vi "get all FPGA CD resources.vi"(7 "Show":T1, 8 "error in (no error)":errorcluster, 11 "Item Ref in":T3 format="%.0x") -> (0 "error out":errorcluster, 2 "resource entries":T2[](array[typedef]) {"FPGA CD Ref" format="%.0x"; "reserver" format="%.0x"}, 3 "Item Ref out":T3 format="%.0x")   [LabVIEW 2016, in "FPGA Resource Manager.lvlib"]
uses:
  FPGA Resource Manager.lvlib
  <vilib>/NI Veristand/Custom Device API/Custom Device Item Ref.ctl
  resource info.ctl
  viz_show.ctl
  <vilib>/NI VeriStand/Custom Device API/Custom Device API.lvlib
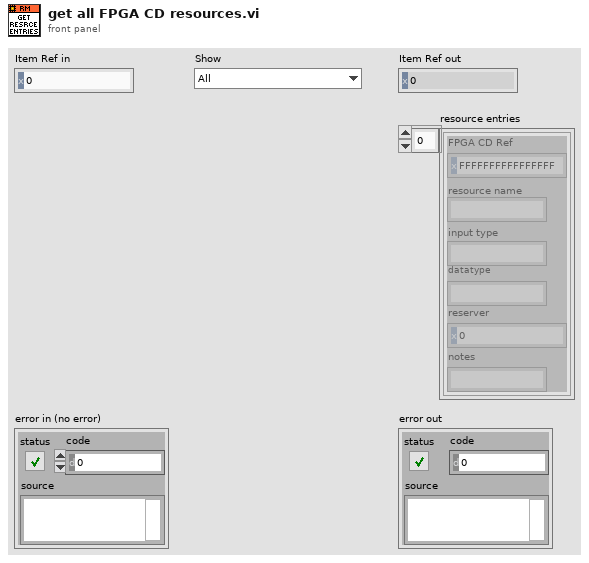
[diagram p1: front panel]
types:
  T1 = typedef "FPGA Resource Manager.lvlib/viz_show.ctl" = enum16{"All", "Mapped", "Unmapped"}
  T2 = typedef "FPGA Resource Manager.lvlib/resource info.ctl" = cluster{"FPGA CD Ref":T3, "resource name":string, "input type":string, "datatype":string, "reserver":T3, "notes":string}
  T3 = typedef "Custom Device API.lvlib/Custom Device Item Ref.ctl" = u64
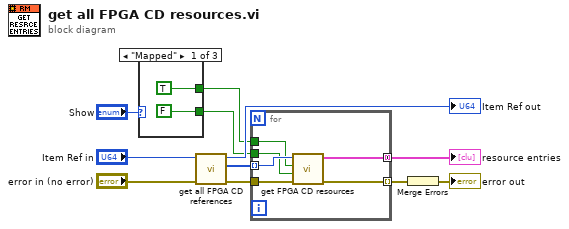
[diagram p0: block diagram]
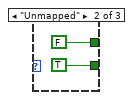
[diagram p2: hidden frame]
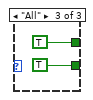
[diagram p3: hidden frame]
diagram:
  n1 = case shown="\"Mapped\"" "Show" {
    tunnel: [TRUE FALSE TRUE] -> w4
    tunnel: [FALSE TRUE TRUE] -> w3
    frame "Mapped" {
    }
    frame "Unmapped" {
    }
    frame "All" {
    }
  }
  n2 = call "get all FPGA CD references.vi"("error in (no error)"="error in (no error)", "Item Ref in"="Item Ref in") -> ("error out"=w8:errorcluster, "RM Server refs out"=w2:T3[], "Item Ref out"=→"Item Ref out":T3)  [unwired: 7 in]
  n3 = for {
    tunnel: w8 -> [w23]
    tunnel: w2 -> [w20] mode=indexing
    tunnel: [w21] -> w10 mode=indexing
    tunnel: [w22] -> w1 mode=concatenating
    tunnel: w4 -> [w19]
    tunnel: w3 -> [w18]
    n4 = call "get FPGA CD resources.vi"("error in (no error)"=w23, "get unmapped?"=w18, "get mapped?"=w19, "Item Ref in"=w20) -> ("error out"=w21:errorcluster, "FPGA CD resources"=w22:T2[])  [unwired: 6 in]
  }
  "resource entries" <- w1
  n5 = Merge Errors(w10) -> (→"error out":errorcluster)
